vi "IsUserLibVI.vi"(11 "ItemPath":path=path "C:/Program Files (x86)/National Instruments/LabVIEW 2023/user.lib/_OpenG.lib/error/error.llb/openg_error.lvlib") -> (3 "IsUserLibVI?":bool)   [LabVIEW 2019, in "DepsWatch.lvlib"]
uses:
  DepsWatch.lvlib
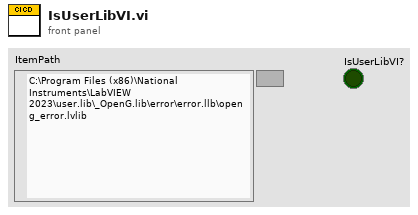
[diagram p1: front panel]
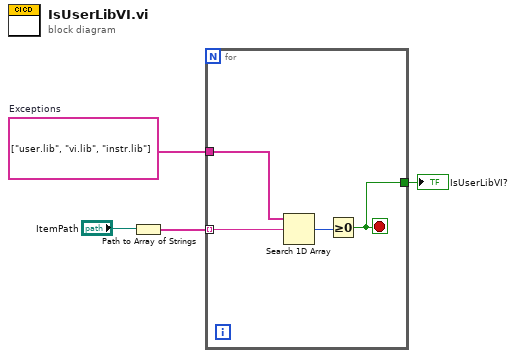
[diagram p0: block diagram]
diagram:
  w2 = string[] ["user.lib", "vi.lib", "instr.lib"]  # Exceptions
  n1 = Path to Array of Strings(0:"ItemPath") -> (2:w3:string[])  [unwired: 1 out]
  n2 = for {
    tunnel: w3 -> [w7] mode=indexing
    tunnel: w2 -> [w8]
    tunnel: [w5] -> w1
    stop <- w5 stop-if-true
    n3 = Search 1D Array(1D array=w8, element=w7) -> (index of element=w6:i32)  [unwired: 1 in]
    n4 = Greater Or Equal To 0?(x=w6) -> (x >= 0?=w5:bool)
  }
  "IsUserLibVI?" <- w1
